vi "Joystick Get.vi"(11 "JoystickDevRef":T1) -> ()   [LabVIEW 2013]
uses:
  <vilib>/Rock Robotics/WPI/Joystick/WPI_JoystickDevRef.ctl
  <vilib>/Rock Robotics/WPI/Joystick/WPI_JoystickDeviceEnum.ctl
  ButtonLayoutDriveJoystick.ctl
  Events.vi
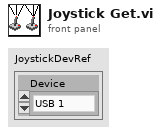
[diagram p1: front panel]
types:
  T1 = typedef "WPI_JoystickDevRef.ctl" = cluster{"Device":T2}
  T2 = typedef "WPI_JoystickDeviceEnum.ctl" = enum16{"USB 1", "USB 2", "USB 3", "USB 4", "Kinect 1", "Kinect 2"}
  T3 = typedef "ButtonLayoutDriveJoystick.ctl" = cluster{"Button 1":bool, "Button 2":bool, "Button 3":bool, "Button 4":bool, "ShiftLow":bool, "ShiftHigh":bool, "Button 7":bool, "Button 8":bool, "Button 9":bool, "Button 10":bool, "Button 11":bool, "Button 12":bool}
  T4 = typedef "WPI_JoystickButtonState.ctl" = cluster{"Button 1":bool, "Button 2":bool, "Button 3":bool, "Button 4":bool, "Button 5":bool, "Button 6":bool, "Button 7":bool, "Button 8":bool, "Button 9":bool, "Button 10":bool, "Button 11":bool, "Button 12":bool}
  T5 = cluster{"axis 1 (x)":dbl, "axis 2 (y)":dbl, "axis 3 (throttle)":dbl, "axis 4":dbl, "axis 5":dbl, "axis 6":dbl}
  T6 = cluster{"Translate":dbl, "Forward Speed":dbl, "Rotate":dbl, "Tank right side":dbl, "axis 5":dbl, "axis 6":dbl}
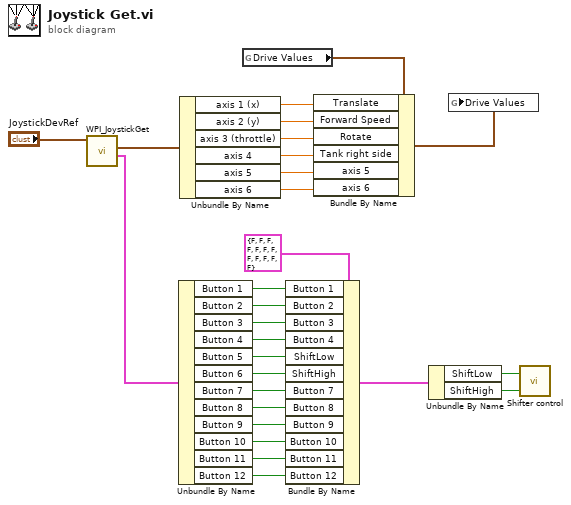
[diagram p0: block diagram]
diagram:
  n1 = call <vilib>:"WPI_JoystickGet.vi"("JoystickDevRef"="JoystickDevRef") -> ("Buttons"=w26:T4, "Axes"=w25:T5)  [unwired: 4 in, 1 out]
  n2 = Unbundle By Name(w26) -> ("Button 1"=w16:bool, "Button 2"=w15:bool, "Button 3"=w14:bool, "Button 4"=w13:bool, "Button 5"=w12:bool, "Button 6"=w11:bool, "Button 7"=w10:bool, "Button 8"=w9:bool, "Button 9"=w8:bool, "Button 10"=w7:bool, "Button 11"=w6:bool, "Button 12"=w5:bool)
  n3 = Unbundle By Name(w25) -> ("axis 1 (x)"=w22:dbl, "axis 2 (y)"=w21:dbl, "axis 3 (throttle)"=w20:dbl, "axis 4"=w19:dbl, "axis 5"=w18:dbl, "axis 6"=w17:dbl)
  n4 = global read "Events.vi" "Drive Values"() -> (w23:T6)
  n5 = Bundle By Name(cluster=T3 {"Button 1"=FALSE, "Button 2"=FALSE, "Button 3"=FALSE, "Button 4"=FALSE, "ShiftLow"=FALSE, "ShiftHigh"=FALSE, "Button 7"=FALSE, "Button 8"=FALSE, "Button 9"=FALSE, "Button 10"=FALSE, "Button 11"=FALSE, "Button 12"=FALSE} ("Buttons"), "Button 1"=w16, "Button 2"=w15, "Button 3"=w14, "Button 4"=w13, "ShiftLow"=w12, "ShiftHigh"=w11, "Button 7"=w10, "Button 8"=w9, "Button 9"=w8, "Button 10"=w7, "Button 11"=w6, "Button 12"=w5) -> (w3:T3)
  n6 = Bundle By Name(cluster=w23, "Translate"=w22, "Forward Speed"=w21, "Rotate"=w20, "Tank right side"=w19, "axis 5"=w18, "axis 6"=w17) -> (w24:T6)
  n7 = Unbundle By Name(w3) -> ("ShiftLow"=w2:bool, "ShiftHigh"=w1:bool)
  n8 = global write "Events.vi" "Drive Values"(w24) -> ()
  n9 = call "Shifter control.vi"("High"=w1, "Low"=w2) -> ()  [unwired: 1 in]
